vi "Delay based on simulated baudrate.vi"(5 "Budrate to simulate":u16, 7 "Number of bytes":i32, 9 "Line Baudrate":u32, 11 "error in":errorcluster) -> (15 "error out":errorcluster)   [LabVIEW 2011]
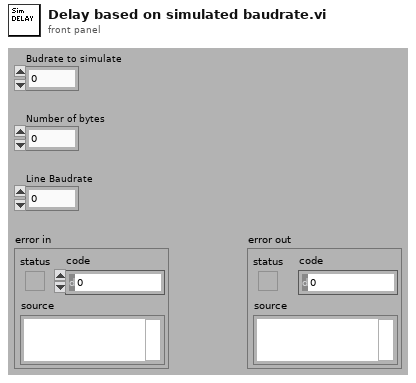
[diagram p1: front panel]
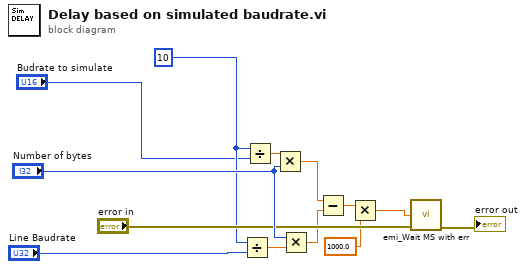
[diagram p0: block diagram]
diagram:
  w2 = 10
  n1 = Divide(x=w2, y="Line Baudrate") -> (x/y=w4:dbl)
  n2 = Divide(x=w2, y="Budrate to simulate") -> (x/y=w3:dbl)
  n3 = Multiply(x=w3, y="Number of bytes") -> (x*y=w5:dbl)
  n4 = Multiply(x="Number of bytes", y=w4) -> (x*y=w6:dbl)
  n5 = Subtract(x=w5, y=w6) -> (x-y=w7:dbl)
  n6 = Multiply(x=w7, y=1000.0) -> (x*y=w10:dbl)
  n7 = call "emi_Wait MS with err.vi"("milliseconds to wait(0)"=w10, "error in (no error)"="error in") -> ("error out"=→"error out":errorcluster)  [unwired: 13 in]
